vi "trafficLight_not_improve.vi"() -> ()   [LabVIEW 2018]
uses:
  color.ctl
  trafficlight.ctl
panel:
  in  "열거형":T1
  in  "light":T2
  out "Red":bool
  out "Orange":bool
  out "Green":bool
  in  "Exit Button":bool
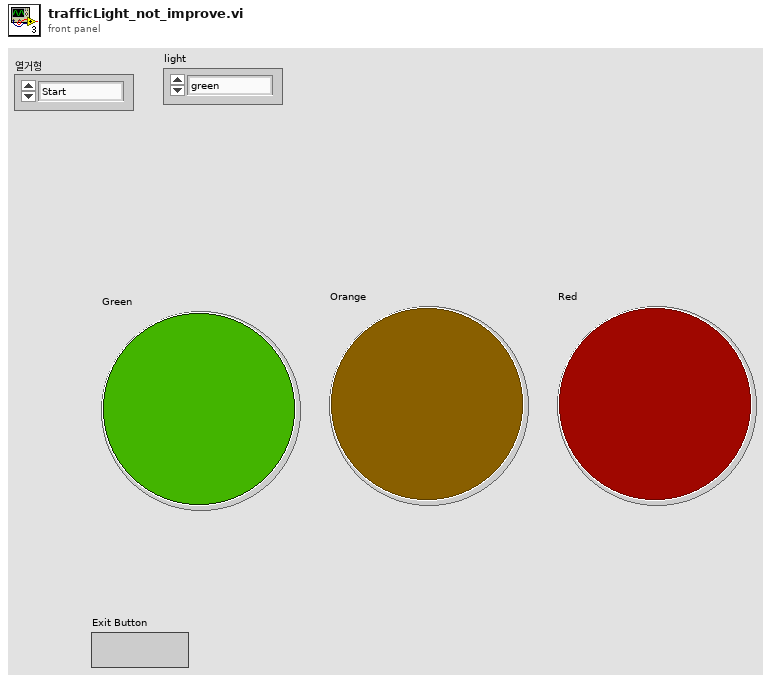
[diagram p1: front panel]
types:
  T1 = typedef "trafficlight.ctl" = enum16{"Start", "LampActivate", "Stop"}
  T2 = typedef "color.ctl" = enum16{"green", "orange", "red"}
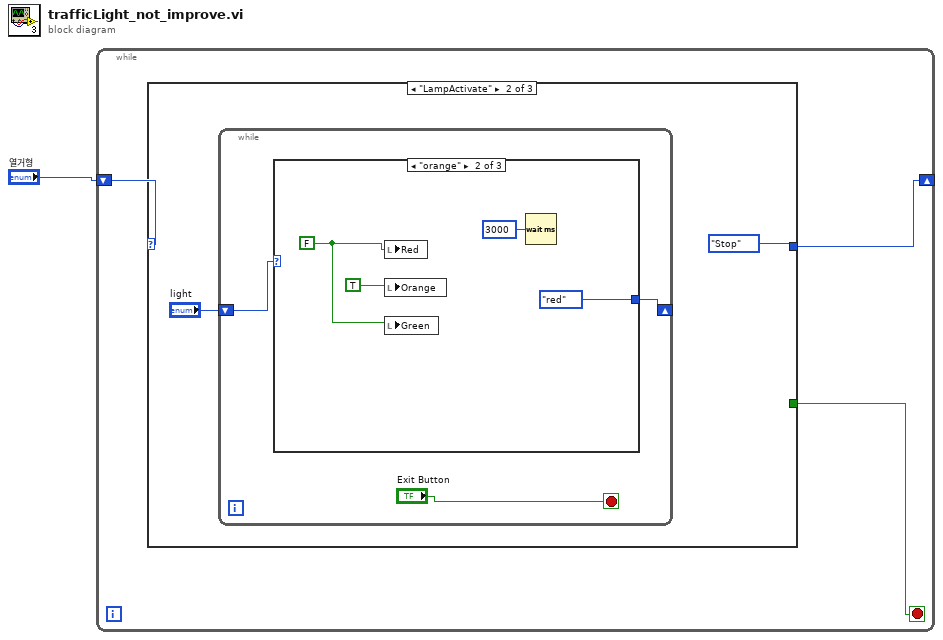
[diagram p0: block diagram]
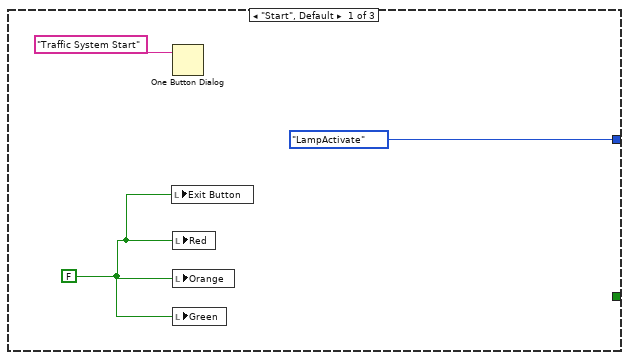
[diagram p2: hidden frame]
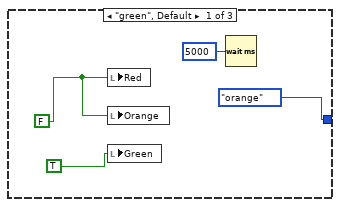
[diagram p3: hidden frame]
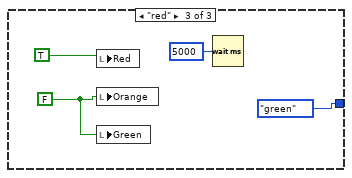
[diagram p4: hidden frame]
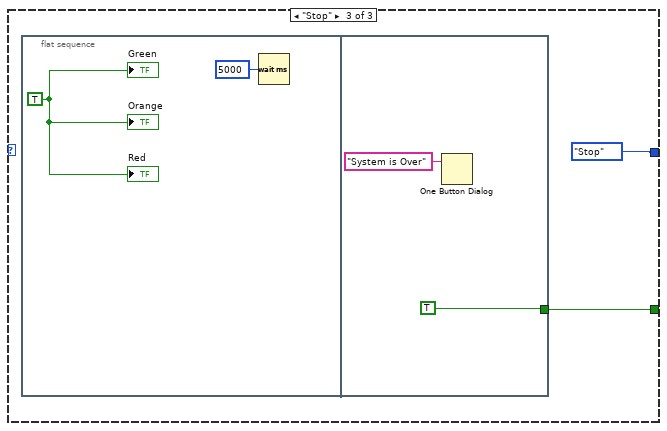
[diagram p5: hidden frame]
diagram:
  n1 = while {
    shift-right: [w3] -> _
    shift-left: "열거형" -> [w4]
    stop <- w2 stop-if-true
    n2 = case shown="\"LampActivate\"" w4 {
      tunnel: [trafficlight."LampActivate" ("열거형") trafficlight."Stop" ("열거형") trafficlight."Stop" ("열거형 2")] -> w3
      tunnel: [_ _ w26] -> w2
      frame "Start", Default {
        w5 = FALSE
        n3 = local write "Exit Button"(w5) -> ()
        n4 = One Button Dialog(message="Traffic System Start" ("메시지")) -> ()  [unwired: 1 in, 1 out]
        n5 = local write "Red"(w5) -> ()
        n6 = local write "Orange"(w5) -> ()
        n7 = local write "Green"(w5) -> ()
      }
      frame "LampActivate" {
        n8 = while {
          shift-right: [w11] -> _
          shift-left: "light" -> [w12]
          stop <- "Exit Button" stop-if-true
          n9 = case shown="\"orange\"" w12 {
            tunnel: [color."orange" ("light 2") color."red" ("light 2") color."green" ("light 2")] -> w11
            frame "green", Default {
              w15 = FALSE
              n10 = local write "Red"(w15) -> ()
              n11 = local write "Orange"(w15) -> ()
              n12 = local write "Green"(TRUE) -> ()
              n13 = Wait (ms)(milliseconds to wait=u32 5000 ("대기 시간 (ms)")) -> ()  [unwired: 1 out]
            }
            frame "orange" {
              w17 = FALSE
              n14 = local write "Red"(w17) -> ()
              n15 = local write "Orange"(TRUE) -> ()
              n16 = local write "Green"(w17) -> ()
              n17 = Wait (ms)(milliseconds to wait=u32 3000 ("대기 시간 (ms)")) -> ()  [unwired: 1 out]
            }
            frame "red" {
              w23 = FALSE
              n18 = local write "Red"(TRUE) -> ()
              n19 = local write "Orange"(w23) -> ()
              n20 = local write "Green"(w23) -> ()
              n21 = Wait (ms)(milliseconds to wait=u32 5000 ("대기 시간 (ms)")) -> ()  [unwired: 1 out]
            }
          }
        }
      }
      frame "Stop" {
        n22 = flat-sequence {
          tunnel: [TRUE] -> w26
          frame #0 {
            w27 = TRUE
            n23 = Wait (ms)(milliseconds to wait=u32 5000 ("대기 시간 (ms)")) -> ()  [unwired: 1 out]
            "Green" <- w27
            "Orange" <- w27
            "Red" <- w27
          }
          frame #1 {
            n24 = One Button Dialog(message="System is Over" ("메시지")) -> ()  [unwired: 1 in, 1 out]
          }
        }
      }
    }
  }
